vi "Pop Header.vi"(8 "error in (no error)":errorcluster, 11 "Header in":refnum<class "Header.lvclass">) -> (0 "error out":errorcluster, 2 "Header Contents":string[](array[string]), 3 "Header out":refnum<class "Header.lvclass">)   [LabVIEW 2018, in "Header.lvclass"]
uses:
  Header.lvclass
  Header.lvclass/Header.ctl
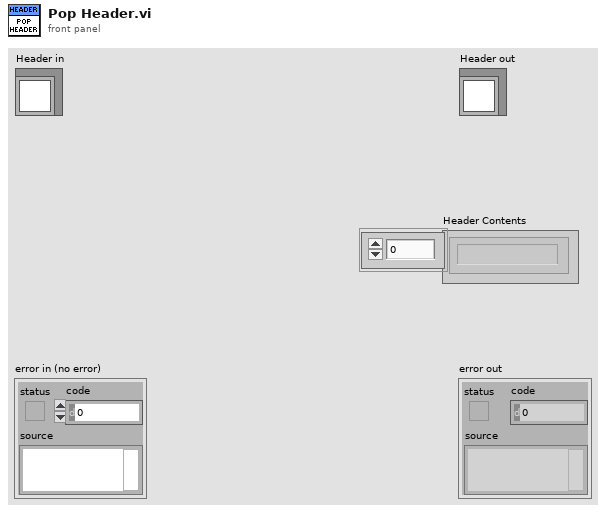
[diagram p1: front panel]
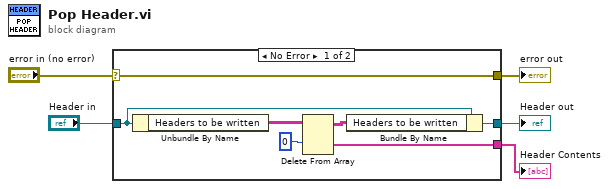
[diagram p0: block diagram]
diagram:
  n1 = case shown="No Error" "error in (no error)" {
    selector: "error in (no error)" -> [w12 w14]
    tunnel: [w12 w14] -> w4
    tunnel: [w8 w13] -> w2
    tunnel: "Header in" -> [w9 w13]
    tunnel: [w6 _] -> w1
    frame No Error {
      n2 = Unbundle By Name(w9) -> ("Headers to be written"=w11:string[][])
      n3 = Delete From Array(array=w11, index (row)=0) -> (deleted portion=w6:string[], array with subset deleted=w7:string[][])  [unwired: 2 in]
      n4 = Bundle By Name(cluster=w9, "Headers to be written"=w7) -> (w8:refnum<class "Header.lvclass">)
    }
    frame Error {
    }
  }
  "error out" <- w4
  "Header out" <- w2
  "Header Contents" <- w1
